vi "CLIENTE GERAL.vi"() -> ()   [LabVIEW 2019]
panel:
  in  "STOP":bool
  in  "NOMES":string[](array[string])
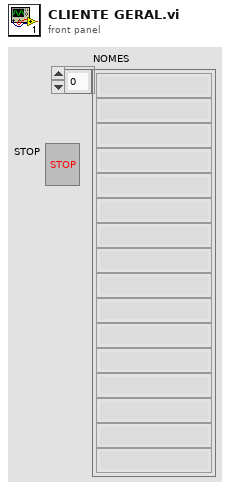
[diagram p1: front panel]
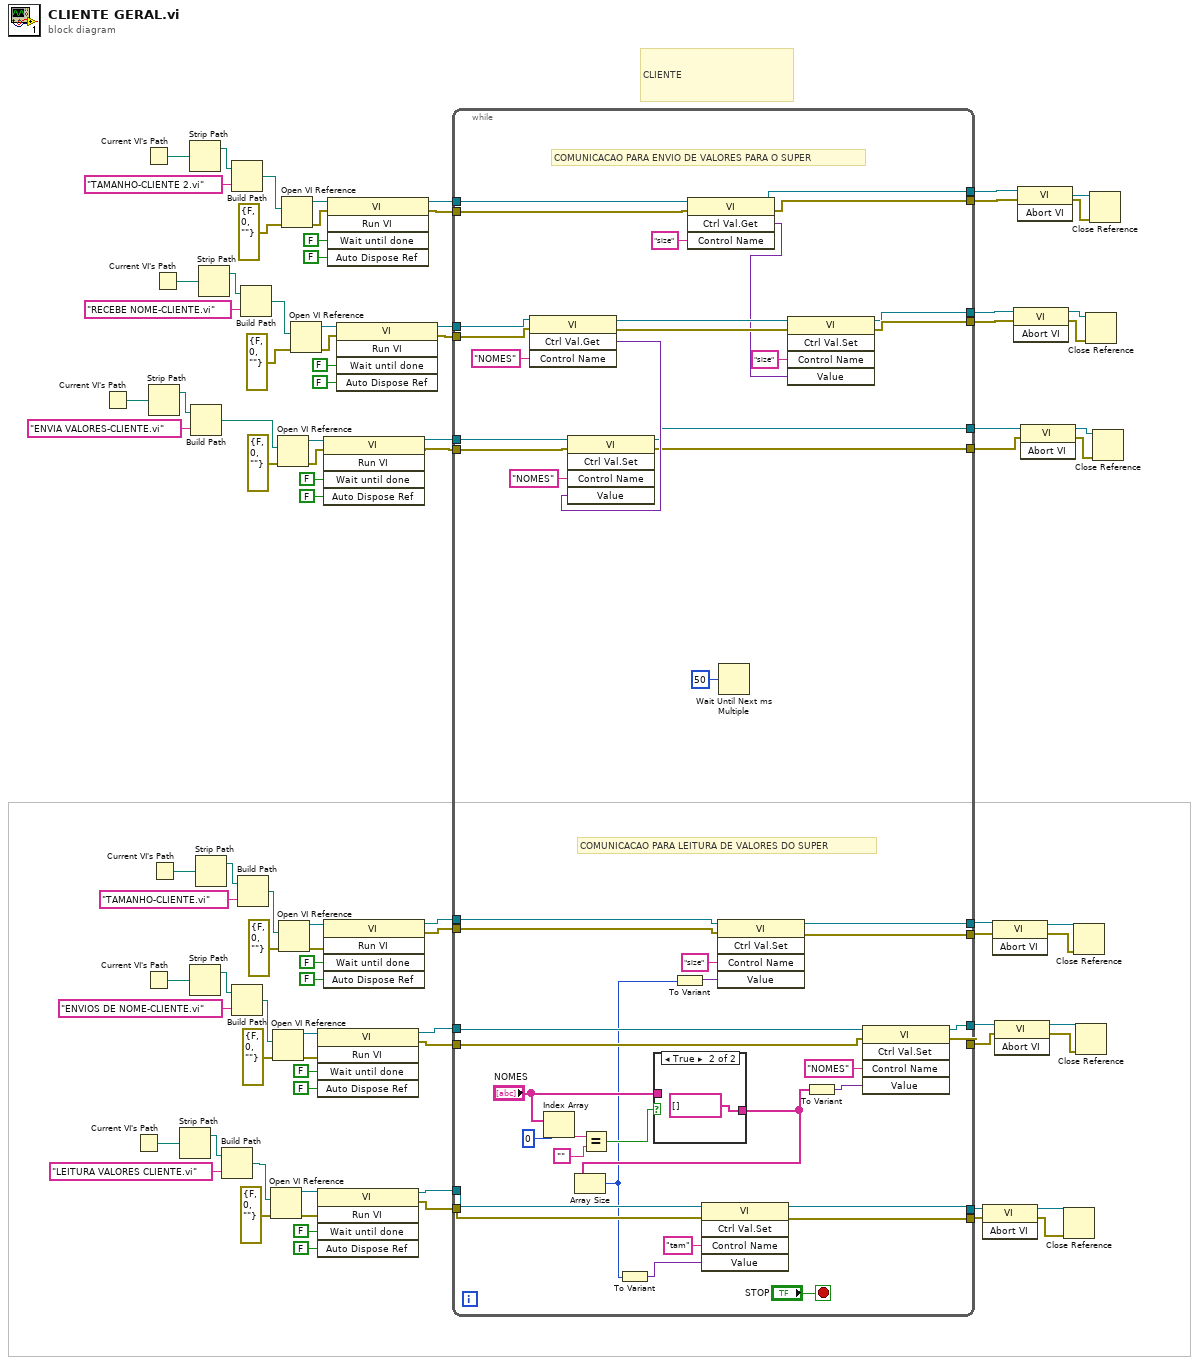
[diagram p0: block diagram]
diagram:
  # "CLIENTE"
  n1 = Current VI's Path() -> (path=w33:path)
  n2 = Current VI's Path() -> (path=w64:path)
  n3 = Current VI's Path() -> (path=w38:path)
  n4 = Current VI's Path() -> (path=w68:path)
  n5 = Strip Path(path=w33) -> (stripped path=w34:path)  [unwired: 1 out]
  n6 = Current VI's Path() -> (path=w55:path)
  n7 = Current VI's Path() -> (path=w30:path)
  n8 = Strip Path(path=w64) -> (stripped path=w63:path)  [unwired: 1 out]
  n9 = Strip Path(path=w38) -> (stripped path=w39:path)  [unwired: 1 out]
  n10 = Strip Path(path=w68) -> (stripped path=w67:path)  [unwired: 1 out]
  n11 = Build Path(base path=w34, name or relative path="ENVIA VALORES-CLIENTE.vi") -> (appended path=w35:path)
  n12 = Strip Path(path=w55) -> (stripped path=w54:path)  [unwired: 1 out]
  n13 = Strip Path(path=w30) -> (stripped path=w31:path)  [unwired: 1 out]
  n14 = Build Path(base path=w63, name or relative path="LEITURA VALORES CLIENTE.vi") -> (appended path=w61:path)
  n15 = Build Path(base path=w39, name or relative path="TAMANHO-CLIENTE 2.vi") -> (appended path=w40:path)
  n16 = Build Path(base path=w67, name or relative path="ENVIOS DE NOME-CLIENTE.vi") -> (appended path=w65:path)
  n17 = Build Path(base path=w54, name or relative path="TAMANHO-CLIENTE.vi") -> (appended path=w52:path)
  n18 = Build Path(base path=w31, name or relative path="RECEBE NOME-CLIENTE.vi") -> (appended path=w32:path)
  n19 = Open VI Reference(vi path=w61, error in (no error)=errorcluster {"status"=FALSE, "code"=0, "source"=""}) -> (vi reference=w85:refnum<vi>, error out=w88:errorcluster)  [unwired: 4 in]
  n20 = Open VI Reference(vi path=w65, error in (no error)=errorcluster {"status"=FALSE, "code"=0, "source"=""}) -> (vi reference=w90:refnum<vi>, error out=w89:errorcluster)  [unwired: 4 in]
  n21 = Open VI Reference(vi path=w35, error in (no error)=errorcluster {"status"=FALSE, "code"=0, "source"=""}) -> (vi reference=w28:refnum<vi>, error out=w29:errorcluster)  [unwired: 4 in]
  n22 = Open VI Reference(vi path=w52, error in (no error)=errorcluster {"status"=FALSE, "code"=0, "source"=""}) -> (vi reference=w60:refnum<vi>, error out=w59:errorcluster)  [unwired: 4 in]
  n23 = Open VI Reference(vi path=w40, error in (no error)=errorcluster {"status"=FALSE, "code"=0, "source"=""}) -> (vi reference=w36:refnum<vi>, error out=w37:errorcluster)  [unwired: 4 in]
  n24 = Open VI Reference(vi path=w32, error in (no error)=errorcluster {"status"=FALSE, "code"=0, "source"=""}) -> (vi reference=w26:refnum<vi>, error out=w27:errorcluster)  [unwired: 4 in]
  n25 = invoke class="VI" method="Run VI"(reference=w90, error in=w89, "Wait until done"=FALSE ("Wait Until Done"), "Auto Dispose Ref"=FALSE ("Auto Dispose Reference")) -> (reference out=w80:refnum<vi>, error out=w79:errorcluster)  [unwired: 1 in, 3 out]
  n26 = invoke class="VI" method="Run VI"(reference=w85, error in=w88, "Wait until done"=FALSE ("Wait Until Done"), "Auto Dispose Ref"=FALSE ("Auto Dispose Reference")) -> (reference out=w74:refnum<vi>, error out=w71:errorcluster)  [unwired: 1 in, 3 out]
  n27 = invoke class="VI" method="Run VI"(reference=w28, error in=w29, "Wait until done"=FALSE ("Wait Until Done"), "Auto Dispose Ref"=FALSE ("Auto Dispose Reference")) -> (reference out=w9:refnum<vi>, error out=w8:errorcluster)  [unwired: 1 in, 3 out]
  n28 = invoke class="VI" method="Run VI"(reference=w60, error in=w59, "Wait until done"=FALSE ("Wait Until Done"), "Auto Dispose Ref"=FALSE ("Auto Dispose Reference")) -> (reference out=w49:refnum<vi>, error out=w48:errorcluster)  [unwired: 1 in, 3 out]
  n29 = invoke class="VI" method="Run VI"(reference=w36, error in=w37, "Wait until done"=FALSE ("Wait Until Done"), "Auto Dispose Ref"=FALSE ("Auto Dispose Reference")) -> (reference out=w5:refnum<vi>, error out=w4:errorcluster)  [unwired: 1 in, 3 out]
  n30 = invoke class="VI" method="Run VI"(reference=w26, error in=w27, "Wait until done"=FALSE ("Wait Until Done"), "Auto Dispose Ref"=FALSE ("Auto Dispose Reference")) -> (reference out=w7:refnum<vi>, error out=w6:errorcluster)  [unwired: 1 in, 3 out]
  n31 = while {
    tunnel: w80 -> [w128]
    tunnel: w79 -> [w127]
    tunnel: [w130] -> w78
    tunnel: [w129] -> w77
    tunnel: w74 -> [w136]
    tunnel: [w134] -> w73
    tunnel: w71 -> [w135]
    tunnel: [w133] -> w72
    tunnel: w49 -> [w117]
    tunnel: w48 -> [w116]
    tunnel: [w115] -> w47
    tunnel: [w114] -> w46
    tunnel: [w103] -> w13
    tunnel: [w102] -> w12
    tunnel: [w101] -> w11
    tunnel: [w100] -> w10
    tunnel: w9 -> [w99]
    tunnel: w8 -> [w98]
    tunnel: w7 -> [w97]
    tunnel: w6 -> [w96]
    tunnel: w5 -> [w95]
    tunnel: w4 -> [w94]
    tunnel: [w92] -> w3
    tunnel: [w91] -> w2
    stop <- "STOP" stop-if-true
    # "COMUNICACAO PARA ENVIO DE VALORES PARA O SUPER"
    # "COMUNICACAO PARA LEITURA DE VALORES DO SUPER"
    n32 = invoke class="VI" method="Ctrl Val.Get"(reference=w97, error in=w96, "Control Name"="NOMES") -> (reference out=w108:refnum<vi>, error out=w107:errorcluster, "Get Control Value Variant"=w93:variant)  [unwired: 1 in, 1 out]
    n33 = Index Array(array="NOMES", index=0) -> (element=w121:string)
    n34 = invoke class="VI" method="Ctrl Val.Set"(reference=w99, error in=w98, "Control Name"="NOMES", "Value"=w93) -> (reference out=w92:refnum<vi>, error out=w91:errorcluster)  [unwired: 1 in, 3 out]
    n35 = Equal?(x=w121, y="") -> (x = y?=w119:bool)
    n36 = case shown="True" w119 {
      tunnel: [w138 string[] [] ("NOMES")] -> w123
      tunnel: "NOMES" -> [w138 _]
      frame False {
      }
      frame True {
      }
    }
    n37 = Array Size(array=w123) -> (size(s)=w111:i32)
    n38 = To Variant(anything=w111) -> (Variant=w131:variant)
    n39 = To Variant(anything=w111) -> (Variant=w112:variant)
    n40 = invoke class="VI" method="Ctrl Val.Get"(reference=w95, error in=w94, "Control Name"="size") -> (reference out=w100:refnum<vi>, error out=w101:errorcluster, "Get Control Value Variant"=w104:variant)  [unwired: 1 in, 1 out]
    n41 = invoke class="VI" method="Ctrl Val.Set"(reference=w136, error in=w135, "Control Name"="tam", "Value"=w131) -> (reference out=w134:refnum<vi>, error out=w133:errorcluster)  [unwired: 1 in, 3 out]
    n42 = invoke class="VI" method="Ctrl Val.Set"(reference=w117, error in=w116, "Control Name"="size", "Value"=w112) -> (reference out=w115:refnum<vi>, error out=w114:errorcluster)  [unwired: 1 in, 3 out]
    n43 = Wait Until Next ms Multiple(millisecond multiple=u32 50) -> ()  [unwired: 1 out]
    n44 = invoke class="VI" method="Ctrl Val.Set"(reference=w108, error in=w107, "Control Name"="size", "Value"=w104) -> (reference out=w102:refnum<vi>, error out=w103:errorcluster)  [unwired: 1 in, 3 out]
    n45 = To Variant(anything=w123) -> (Variant=w125:variant)
    n46 = invoke class="VI" method="Ctrl Val.Set"(reference=w128, error in=w127, "Control Name"="NOMES", "Value"=w125) -> (reference out=w130:refnum<vi>, error out=w129:errorcluster)  [unwired: 1 in, 3 out]
  }
  n47 = invoke class="VI" method="Abort VI"(reference=w73, error in=w72) -> (reference out=w75:refnum<vi>, error out=w70:errorcluster)  [unwired: 1 in, 1 out]
  n48 = invoke class="VI" method="Abort VI"(reference=w47, error in=w46) -> (reference out=w51:refnum<vi>, error out=w50:errorcluster)  [unwired: 1 in, 1 out]
  n49 = invoke class="VI" method="Abort VI"(reference=w78, error in=w77) -> (reference out=w76:refnum<vi>, error out=w69:errorcluster)  [unwired: 1 in, 1 out]
  n50 = invoke class="VI" method="Abort VI"(reference=w12, error in=w13) -> (reference out=w42:refnum<vi>, error out=w43:errorcluster)  [unwired: 1 in, 1 out]
  n51 = invoke class="VI" method="Abort VI"(reference=w10, error in=w11) -> (reference out=w44:refnum<vi>, error out=w45:errorcluster)  [unwired: 1 in, 1 out]
  n52 = invoke class="VI" method="Abort VI"(reference=w3, error in=w2) -> (reference out=w41:refnum<vi>, error out=w1:errorcluster)  [unwired: 1 in, 1 out]
  n53 = Close Reference(reference=w75, error in (no error)=w70) -> ()  [unwired: 1 out]
  n54 = Close Reference(reference=w51, error in (no error)=w50) -> ()  [unwired: 1 out]
  n55 = Close Reference(reference=w76, error in (no error)=w69) -> ()  [unwired: 1 out]
  n56 = Close Reference(reference=w42, error in (no error)=w43) -> ()  [unwired: 1 out]
  n57 = Close Reference(reference=w44, error in (no error)=w45) -> ()  [unwired: 1 out]
  n58 = Close Reference(reference=w41, error in (no error)=w1) -> ()  [unwired: 1 out]
